vi "Apply.vi"(8 "error in":errorcluster, 11 "IMAQdx Base Configure Strategy in":refnum<class "IMAQdx Base Configure Strategy.lvclass">) -> (0 "error out":errorcluster, 3 "IMAQdx Base Configure Strategy out":refnum<class "IMAQdx Base Configure Strategy.lvclass">)   [LabVIEW 2025, in "IMAQdx Base Configure Strategy.lvclass"]
uses:
  IMAQdx Base Configure Strategy.lvclass
  IMAQdx Base Configure Strategy.lvclass/IMAQdx Base Configure Strategy.ctl
  <vilib>/vision/driver/NI_Vision_Acquisition_Software.lvlib
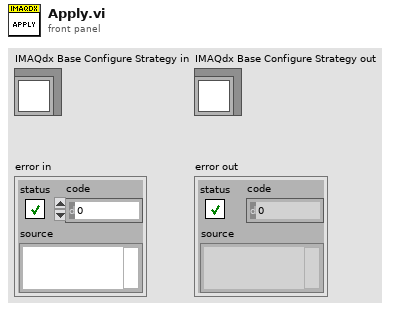
[diagram p1: front panel]
types:
  T1 = typedef "IMAQdx.ctl" = refnum<k21>
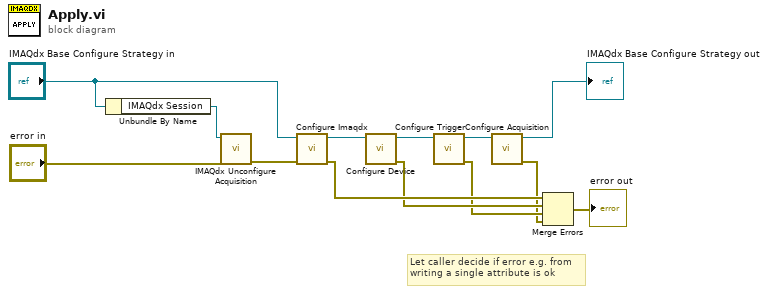
[diagram p0: block diagram]
diagram:
  # "Let caller decide if error e.g. from\nwriting a single attribute is ok"
  n1 = Unbundle By Name("IMAQdx Base Configure Strategy in") -> ("IMAQdx Session"=w11:T1)
  n2 = call <vilib>:"IMAQdx Unconfigure Acquisition.vi"("error in"="error in", "Session In"=w11) -> ("error out"=w12:errorcluster)  [unwired: 8 in, 1 out]
  n3 = call-dynamic "Configure Imaqdx.vi"("error in"=w12, "IMAQdx Base Configure Strategy in"="IMAQdx Base Configure Strategy in") -> ("error out"=w5:errorcluster, "IMAQdx Base Configure Strategy out"=w7:refnum<class "IMAQdx Base Configure Strategy.lvclass">)  [unwired: 8 in]
  n4 = call-dynamic "Configure Device.vi"("IMAQdx Base Configure Strategy in"=w7) -> ("error out"=w4:errorcluster, "IMAQdx Base Configure Strategy out"=w9:refnum<class "IMAQdx Base Configure Strategy.lvclass">)  [unwired: 9 in]
  n5 = call-dynamic "Configure Trigger.vi"("IMAQdx Base Configure Strategy in"=w9) -> ("error out"=w3:errorcluster, "IMAQdx Base Configure Strategy out"=w10:refnum<class "IMAQdx Base Configure Strategy.lvclass">)  [unwired: 9 in]
  n6 = call-dynamic "Configure Acquisition.vi"("IMAQdx Base Configure Strategy in"=w10) -> ("error out"=w2:errorcluster, "IMAQdx Base Configure Strategy out"=→"IMAQdx Base Configure Strategy out":refnum<class "IMAQdx Base Configure Strategy.lvclass">)  [unwired: 9 in]
  n7 = Merge Errors(w5, w4, w3, w2) -> (→"error out":errorcluster)
